vi "KEITHLEY-24XX-I-V.vi"() -> ()   [LabVIEW 2020]
uses:
  <instrlib>/Keithley 24XX/Public/Data/Read (Single Point).vi
  <instrlib>/Keithley 24XX/Keithley 24XX.lvlib
panel:
  in  "Serial Configuration":T1={"Baud Rate"=9600, "Parity"=0, "Data Bits"=8, "Stop Bits"=10, "Flow Control"=0} {"Flow Control" items=["None", "XON/XOFF", "RTS/CTS", "XON/XOFF & RTS/CTS", "DTR/DSR", "XON/XOFF & DTR/DSR"]; "Stop Bits" items=["1.0"=10, "1.5"=15, "2.0"=20]; "Data Bits" items=["7"=7, "8"=8]; "Parity" items=["None", "Odd", "Even", "Mark", "Space"]; "Baud Rate" items=["300"=300, "600"=600, "1200"=1200, "2400"=2400, "4800"=4800, "9600"=9600, "19200"=19200]}
  in  "VISA resource name":refnum<visa-resource-name>
  out "Table Control":string[][](table)
  out "XY Graph 2":cluster{"ÇIKIÞ VOLTAJI":dbl[], "AKIM":dbl[]}(graph)
  in  "stop":bool
  out "AKIM":dbl[](array[numeric])
  in  "Step delay time":u32
  in  "Max current value":dbl=0.1
  out "TERÝM SAYISI":dbl
  out "ÇIKIÞ VOLTAJI":dbl[](array[numeric])
  in  "Final voltage":dbl
  in  "Increment amount":dbl
  in  "Initial voltage":dbl
  in  "4W":bool=TRUE
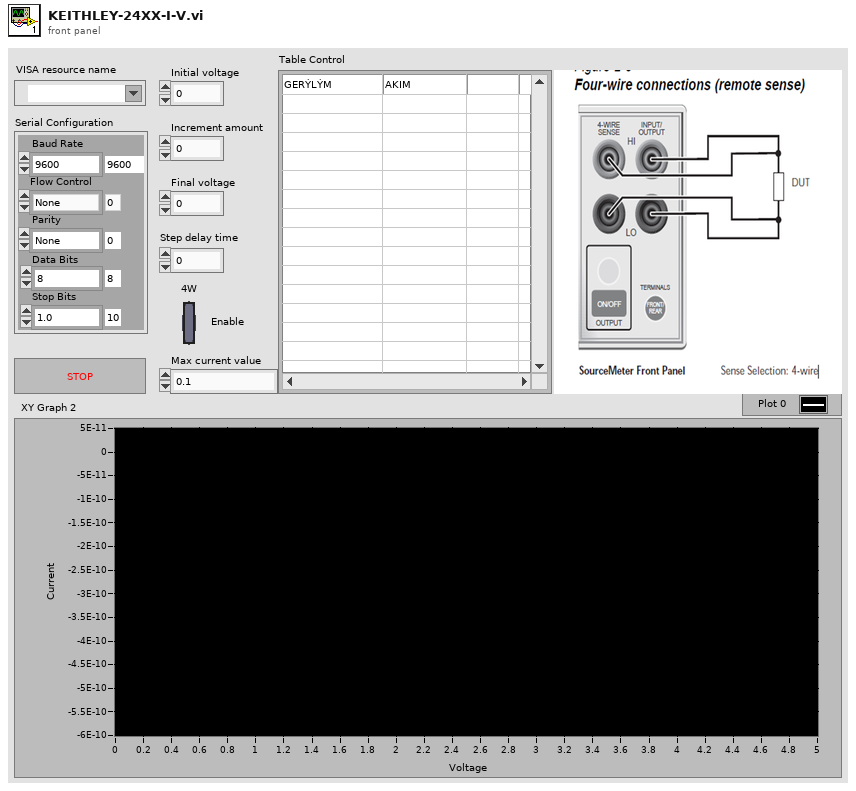
[diagram p1: front panel]
types:
  T1 = cluster{"Baud Rate":u32, "Parity":u16, "Data Bits":u16, "Stop Bits":u16, "Flow Control":u16}
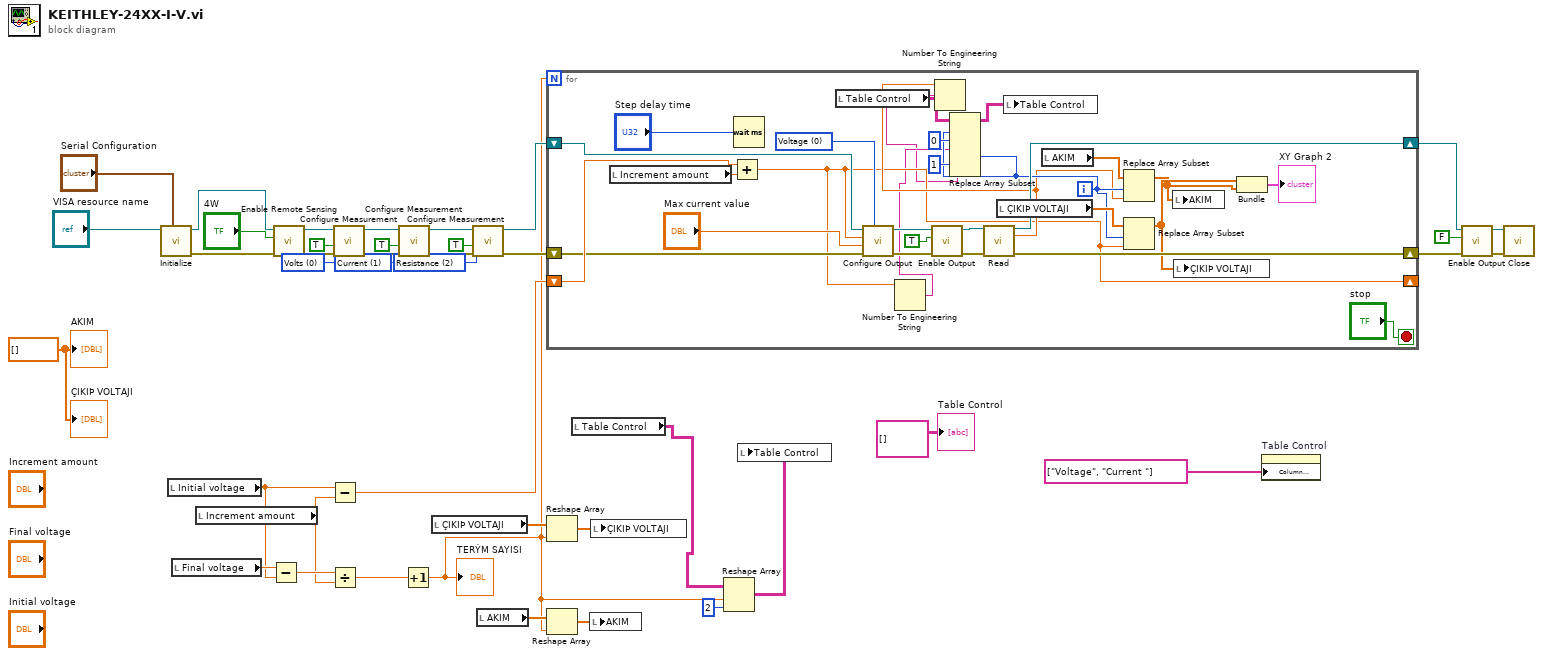
[diagram p0: block diagram]
diagram:
  w12 = u16 2 items=["Volts", "Current", "Resistance"] ("Function (0: Volts)")
  w13 = u16 1 items=["Volts", "Current", "Resistance"] ("Function (0: Volts)")
  w14 = u16 0 items=["Volts", "Current", "Resistance"] ("Function (0: Volts)")
  w17 = dbl[] []
  n1 = call <instrlib>:"Initialize.vi"("Serial Configuration"="Serial Configuration", "VISA resource name"="VISA resource name") -> ("error out"=w40:errorcluster, "VISA resource name out"=w41:refnum<visa-resource-name>)  [unwired: 8 in]
  n2 = local read "Initial voltage"() -> (w34:dbl)
  n3 = local read "Final voltage"() -> (w37:dbl)
  n4 = local read "Increment amount"() -> (w33:dbl)
  n5 = Subtract(x=w37, y=w34) -> (x-y=w36:dbl)
  n6 = call <instrlib>:"Enable Remote Sensing.vi"("error in (no error)"=w40, "Enable Remote Sensing (T: Enable)"="4W", "VISA resource name"=w41) -> ("error out"=w30:errorcluster, "VISA resource name out"=w31:refnum<visa-resource-name>)  [unwired: 7 in]
  n7 = Subtract(x=w34, y=w33) -> (x-y=w25:dbl)
  n8 = Divide(x=w36, y=w33) -> (x/y=w35:dbl)
  n9 = call <instrlib>:"Configure Measurement.vi"("error in (no error)"=w30, "Enable Auto Range (T:Enable)"=TRUE, "Function (0: Volts)"=w14, "VISA resource name"=w31) -> ("error out"=w28:errorcluster, "VISA resource name out"=w29:refnum<visa-resource-name>)  [unwired: 6 in]
  n10 = call <instrlib>:"Configure Measurement.vi"("error in (no error)"=w28, "Enable Auto Range (T:Enable)"=TRUE, "Function (0: Volts)"=w13, "VISA resource name"=w29) -> ("error out"=w26:errorcluster, "VISA resource name out"=w27:refnum<visa-resource-name>)  [unwired: 6 in]
  n11 = Increment(x=w35) -> (x+1=w5:dbl)
  "TERÝM SAYISI" <- w5
  n12 = local read "ÇIKIÞ VOLTAJI"() -> (w39:dbl[])
  n13 = call <instrlib>:"Configure Measurement.vi"("error in (no error)"=w26, "Enable Auto Range (T:Enable)"=TRUE, "Function (0: Volts)"=w12, "VISA resource name"=w27) -> ("error out"=w23:errorcluster, "VISA resource name out"=w24:refnum<visa-resource-name>)  [unwired: 6 in]
  n14 = local read "AKIM"() -> (w15:dbl[])
  n15 = for {
    N: w5 -> [_]
    shift-right: [w59] -> w18
    shift-left: w24 -> [w65]
    shift-right: [w58] -> w21
    shift-left: w23 -> [w64]
    shift-right: [w44] -> _
    shift-left: w25 -> [w67]
    i -> [w46]
    stop <- "stop" stop-if-true
    w56 = u16 0 items=["Voltage", "Current"] ("Source Mode  (0: Voltage)")
    n16 = local read "Increment amount"() -> (w69:dbl)
    n17 = Add(x=w67, y=w69) -> (x+y=w44:dbl)
    n18 = Wait (ms)(milliseconds to wait="Step delay time") -> ()  [unwired: 1 out]
    n19 = local read "Table Control"() -> (w50:string[][])
    n20 = call <instrlib>:"Configure Output.vi"("Source Mode  (0: Voltage)"=w56, "error in (no error)"=w64, "Compliance  Level (0.1)"="Max current value", "Output Level (0)"=w44, "VISA resource name"=w65) -> ("error out"=w62:errorcluster, "VISA resource name out"=w63:refnum<visa-resource-name>)  [unwired: 5 in]
    n21 = Number To Engineering String(4:w44) -> (0:w43:string)  [unwired: 3 in]
    n22 = call <instrlib>:"Enable Output.vi"("error in (no error)"=w62, "Enable Output (T: Enable)"=TRUE, "VISA resource name"=w63) -> ("error out"=w61:errorcluster, "VISA resource name out"=w60:refnum<visa-resource-name>)  [unwired: 7 in]
    n23 = call-poly <instrlib>:"Read.vi"("VISA resource name"=w60, "error in (no error)"=w61) -> ("VISA resource name out"=w59:refnum<visa-resource-name>, "Current"=w45:sgl, "error out"=w58:errorcluster)  [unwired: 7 in, 4 out]
    n24 = Number To Engineering String(4:w45) -> (0:w42:string)  [unwired: 3 in]
    n25 = Replace Array Subset(array=w50, new element #1=w43, index (row) #1=w46, index (col) #1=0 ("disabled index (col)"), new element #2=w42, index (row) #2=w46, index (col) #2=1 ("index (col)")) -> (w49:string[][])
    n26 = local read "ÇIKIÞ VOLTAJI"() -> (w68:dbl[])
    n27 = local write "Table Control"(w49) -> ()
    n28 = local read "AKIM"() -> (w55:dbl[])
    n29 = Replace Array Subset(array=w55, new element=w45, index=w46) -> (w52:dbl[])
    n30 = Replace Array Subset(array=w68, new element=w44, index=w46) -> (w53:dbl[])
    n31 = local write "AKIM"(w52) -> ()
    n32 = local write "ÇIKIÞ VOLTAJI"(w53) -> ()
    n33 = Bundle("ÇIKIÞ VOLTAJI"=w53, "AKIM"=w52) -> (→"XY Graph 2":cluster{"ÇIKIÞ VOLTAJI":dbl[], "AKIM":dbl[]})  [unwired: 1 in]
  }
  n34 = Reshape Array(w39, w5) -> (w38:dbl[])
  n35 = Reshape Array(w15, w5) -> (w16:dbl[])
  n36 = local read "Table Control"() -> (w7:string[][])
  n37 = local write "AKIM"(w16) -> ()
  n38 = local write "ÇIKIÞ VOLTAJI"(w38) -> ()
  n39 = Reshape Array(w7, w5, 2 ("dimension size")) -> (w6:string[][])
  n40 = local write "Table Control"(w6) -> ()
  n41 = property on="Table Control" class="Tbl (strict)"("Column Headers[]"=string[] ["Voltage", "Current "] ("Row Header Strings[]")) -> ()  [unwired: 2 in, 2 out]
  n42 = call <instrlib>:"Enable Output.vi"("error in (no error)"=w21, "Enable Output (T: Enable)"=FALSE, "VISA resource name"=w18) -> ("error out"=w20:errorcluster, "VISA resource name out"=w19:refnum<visa-resource-name>)  [unwired: 7 in]
  n43 = call <instrlib>:"Close.vi"("error in (no error)"=w20, "VISA resource name"=w19) -> ()  [unwired: 9 in, 1 out]
  "ÇIKIÞ VOLTAJI" <- w17
  "AKIM" <- w17
  "Table Control" <- string[][] [] ("Table Control")
